vi "gfitsio-read-key-logical.vi"(7 "keyname":string, 8 "error in (no error)":errorcluster, 9 "default value":bool, 11 "gfits refnum":T1) -> (0 "error out":errorcluster, 1 "comment":string, 2 "value":bool, 3 "dup gfits refnum":T1)   [LabVIEW 2011, in "gfitsio.lvlib"]
doc: "Return the specified keyword. <B>default value</B> specifies the desired returned data type of the keyword value. Data type conversion will be performed for numeric values if the keyword value does not have the same data type. If the keyword does not exist or an error occurs <B>value</B> will be equal to <B>default value</B>."
uses:
  gfitsio.lvlib
  gfitsio-refnum.ctl
  cfitsio-hdutypes.ctl
  gfitsio.dll
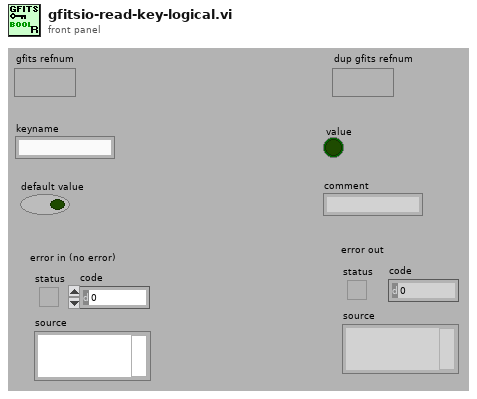
[diagram p1: front panel]
types:
  T1 = typedef "gfitsio.lvlib/gfitsio-refnum.ctl" = refnum<k1>
  T2 = typedef "gfitsio.lvlib/cfitsio-hdutypes.ctl" = i32
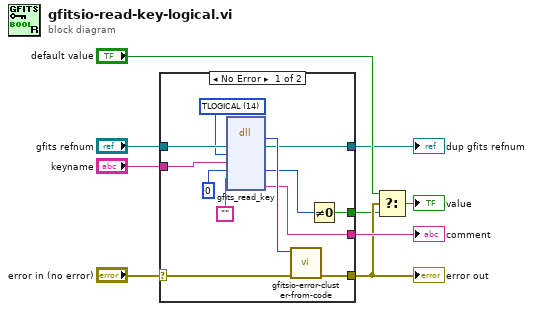
[diagram p0: block diagram]
diagram:
  n1 = case shown="No Error" "error in (no error)" {
    selector: "error in (no error)" -> [w20 w23]
    tunnel: [w19 w23] -> w3
    tunnel: "gfits refnum" -> [w17 w22]
    tunnel: [w18 w22] -> w1
    tunnel: "keyname" -> [w15 _]
    tunnel: [w10 _] -> w2
    tunnel: [w12 _] -> w4
    frame No Error {
      w16 = T2 14 items=["TBIT"=1, "TBYTE  (U8)"=11, "TSBYTE  (I8)"=12, "TLOGICAL"=14, "TSTRING"=16, "TUSHORT  (U16)"=20, "TSHORT  (I16)"=21, "TUINT"=31, "TULONG  (U32)"=40, "TLONG  (I32)"=41, "TFLOAT  (SGL)"=42, "TLONGLONG  (I64)"=81, "TDOUBLE"=82, "TCOMPLEX  (CSG)"=83, "TDOUBLECOMPLEX  (CDB)"=163] ("cfitsio datatype")
      n2 = dll-call lib="C:/BonOMM/BonOMM-SAOMM/SubVIs/gfitsio/gfitsio.dll" fn="gfits_read_key"("gfits refnum"=w17, "datatype"=w16, "keyname"=w15, "value"=u8 0, "units"="") -> (w21:i32, "gfits refnum"=w18:T1, "value"=w13:u8, "comment"=w12:string)  [unwired: 7 in, 2 out]
      n3 = call "gfitsio-error-cluster-from-code.vi"("error in (no error)"=w20, "error code"=w21) -> ("error out"=w19:errorcluster)  [unwired: 9 in]
      n4 = Not Equal To 0?(x=w13) -> (x != 0?=w10:bool)
    }
    frame Error {
    }
  }
  "error out" <- w3
  "dup gfits refnum" <- w1
  "comment" <- w4
  n5 = Select(t="default value", s=w3, f=w2) -> (s? t:f=→"value":bool)
